vi "故障码字段定义.vi"(11 "故障代码":u16) -> (3 "data":T1)   [LabVIEW 2016, in "斯坦道CODMn新电路板.lvlib"]
uses:
  Alarm interface/Alarm interface.lvlib
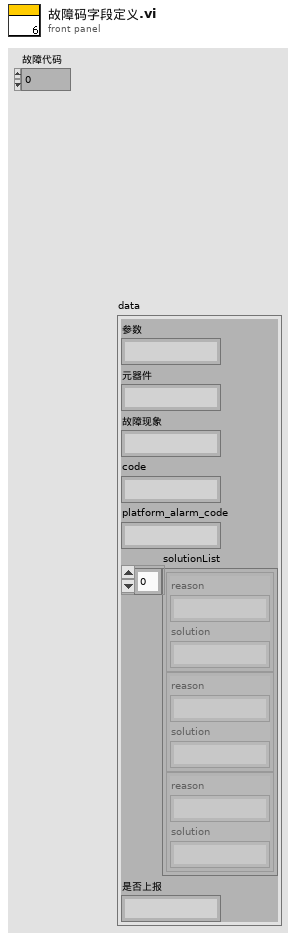
[diagram p1: front panel]
types:
  T1 = typedef "Alarm interface.lvlib/报警短信语音交互.ctl" = cluster{"参数":string, "元器件":string, "故障现象":string, "code":string, "platform_alarm_code":string, "solutionList":cluster{"reason":string, "solution":string}[], "是否上报":string}
  T2 = typedef "Alarm interface.lvlib/map in.ctl" = cluster{"name":string, "CN":string, "FirmwareVersion":string, "code":string}
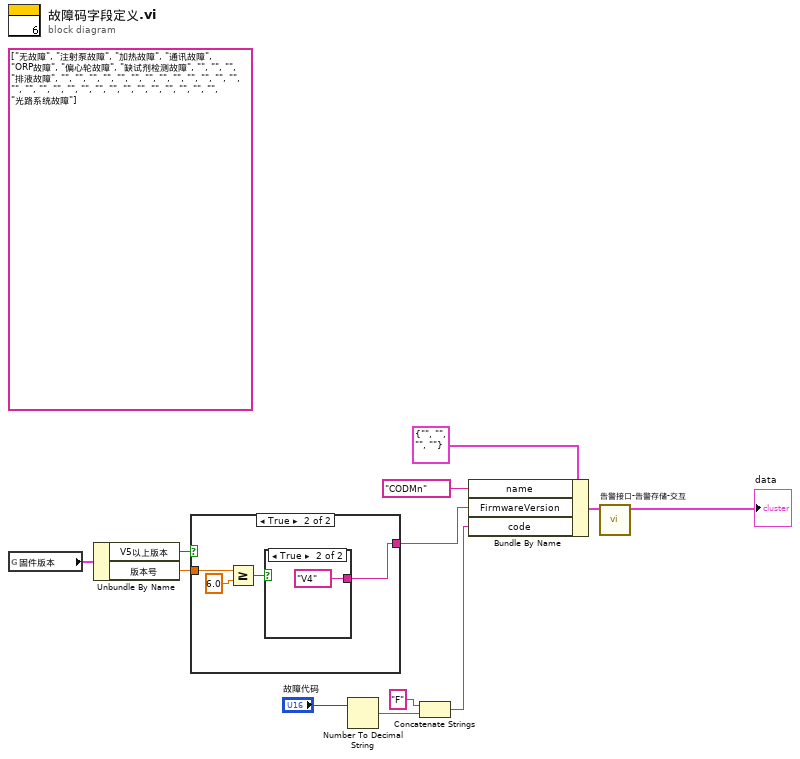
[diagram p0: block diagram]
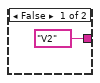
[diagram p2: hidden frame]
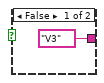
[diagram p3: hidden frame]
diagram:
  (unwired) string[] ["无故障", "注射泵故障", "加热故障", "通讯故障", "ORP故障", "偏心轮故障", "缺试剂检测故障", "", "", "", "排液故障", "", "", "", "", "", "", "", "", "", "", "", "", "", "", "", "", "", "", "", "", "", "", "", "", "", "", "", "", "光路系统故障"]
  n1 = global read "VARCODMn全局变量.vi" "固件版本"() -> (w6:cluster{"V5以上版本":bool, "版本号":dbl})
  n2 = Unbundle By Name(w6) -> ("V5以上版本"=w5:bool, "版本号"=w4:dbl)
  n3 = case shown="True" w5 {
    tunnel: ["V2" ("equipVersion") w17] -> w3
    tunnel: w4 -> [_ w15]
    frame False {
    }
    frame True {
      n4 = Greater Or Equal?(x=w15, y=6.0) -> (x >= y?=w14:bool)
      n5 = case shown="True" w14 {
        tunnel: ["V3" ("equipVersion") "V4" ("equipVersion")] -> w17
        frame False {
        }
        frame True {
        }
      }
    }
  }
  n6 = Number To Decimal String(number="故障代码") -> (decimal integer string=w11:string)  [unwired: 1 in]
  n7 = Concatenate Strings("F" ("字符串"), w11) -> (w8:string)
  n8 = Bundle By Name(cluster=T2 {"name"="", "CN"="", "FirmwareVersion"="", "code"=""} ("map in"), "name"="CODMn" ("componentParent"), "FirmwareVersion"=w3, "code"=w8) -> (w1:T2)
  n9 = call "告警接口-告警存储-交互.vi"("map in"=w1) -> ("data"=→"data":T1)  [unwired: 10 in]
